vi "Check Status.vi"(8 "error in (no error)":errorcluster, 11 "Spectrometer Digikröm in":refnum<class "Spectrometer Digikröm.lvclass">) -> (0 "error out":errorcluster, 1 "Status":string, 2 "Ready?":bool, 3 "Spectrometer Digikröm out":refnum<class "Spectrometer Digikröm.lvclass">)   [LabVIEW 2023, in "Spectrometer Digikröm.lvclass"]
doc: "(Dynamic) Check if the instrument is powered on and update its member fields with the instrument's current status. Optionally return a text status message."
uses:
  Utility Classes/Scannable/Scannable.lvclass
  Digikrom DK24x/Digikrom DK24x.lvlib
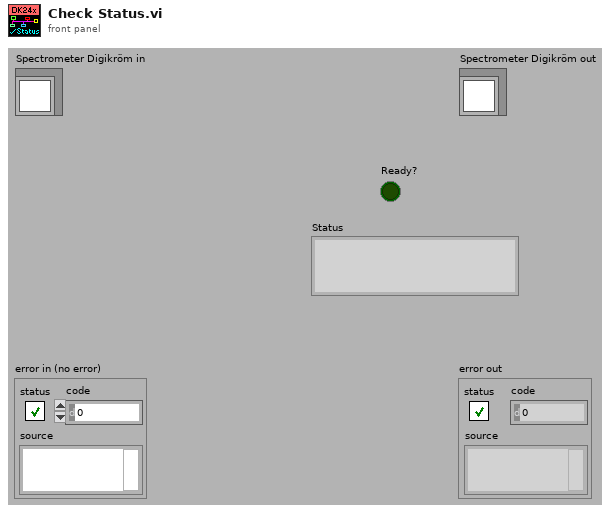
[diagram p1: front panel]
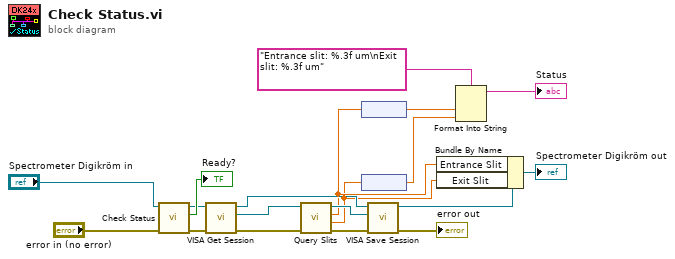
[diagram p0: block diagram]
diagram:
  n1 = call-parent "Check Status.vi"("error in (no error)"="error in (no error)", "Instrument in"="Spectrometer Digikröm in") -> ("error out"=w15:errorcluster, "Ready?"=→"Ready?":bool, "Instrument out"=w16:refnum<class "Spectrometer Digikröm.lvclass">)  [unwired: 6 in, 1 out]
  n2 = call-dynamic "VISA Get Session.vi"("error in (no error)"=w15, "Instrument.lvclass in"=w16) -> ("error out"=w2:errorcluster, "VISA Resource Name"=w1:refnum<visa-resource-name>, "Instrument.lvclass out"=w13:refnum<class "Spectrometer Digikröm.lvclass">)  [unwired: 7 out]
  n3 = call "Query Slits.vi"("error in (no error)"=w2, "VISA resource name"=w1) -> ("error out"=w12:errorcluster, "CURRENT S2 WIDTH"=w7:dbl[unit], "CURRENT S1 WIDTH"=w8:dbl[unit], "VISA resource name out"=w14:refnum<visa-resource-name>)  [unwired: 6 out]
  n4 = node(w8) -> (w5:dbl)
  n5 = node(w7) -> (w4:dbl)
  n6 = call-dynamic "VISA Save Session.vi"("error in (no error)"=w12, "VISA Resource Name"=w14, "Instrument.lvclass in"=w13) -> ("error out"=→"error out":errorcluster, "Instrument.lvclass out"=w10:refnum<class "Spectrometer Digikröm.lvclass">)  [unwired: 7 out]
  n7 = Bundle By Name(cluster=w10, "Entrance Slit"=w8, "Exit Slit"=w7) -> (→"Spectrometer Digikröm out":refnum<class "Spectrometer Digikröm.lvclass">)
  n8 = Format Into String(format string="Entrance slit: %.3f um\nExit slit: %.3f um", w5, w4) -> (resulting string=→"Status":string)  [unwired: 2 in, 1 out]
